vi "Read Measurement (FM Demodulation).vi"(0 "VISA resource name":refnum<visa-resource-name>, 11 "error in (no error)":errorcluster) -> (2 "Carrier Power (dBm)":dbl[](array[numeric]), 3 "Modulation Rate (Hz)":dbl[](array[numeric]), 4 "VISA resource name out":refnum<visa-resource-name>, 6 "Frequency Deviation (Hz)":dbl[](array[numeric]), 8 "SINAD (dB)":dbl[](array[numeric]), 10 "THD (dB)":dbl[](array[numeric]), 14 "Carrier Frequency Offset (Hz)":dbl[](array[numeric]), 15 "error out":errorcluster)   [LabVIEW 2022 SP3, in "Agilent N934X Series.lvlib"]
doc: "Reads the measurement result from the spectrum analyzer(FM Demodulation Measurement).\n\nNotes:\n\n(1) This VI is only applicable for N9321C, N9322C, N9323C, N9324C models.\n(2) User must use <B>Configure Measurement Type.vi</B> to change the mode to <B>Frequency Modulation</B> before using this VI."
uses:
  <instrlib>/Agilent N934X Series/Agilent N934X Series.lvlib
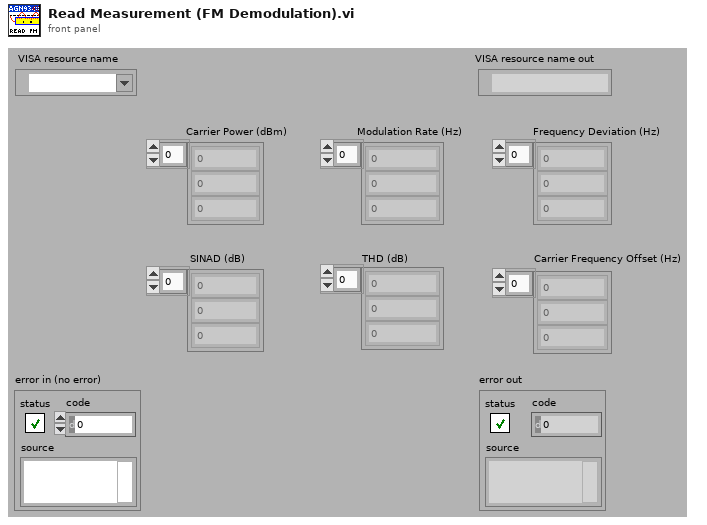
[diagram p1: front panel]
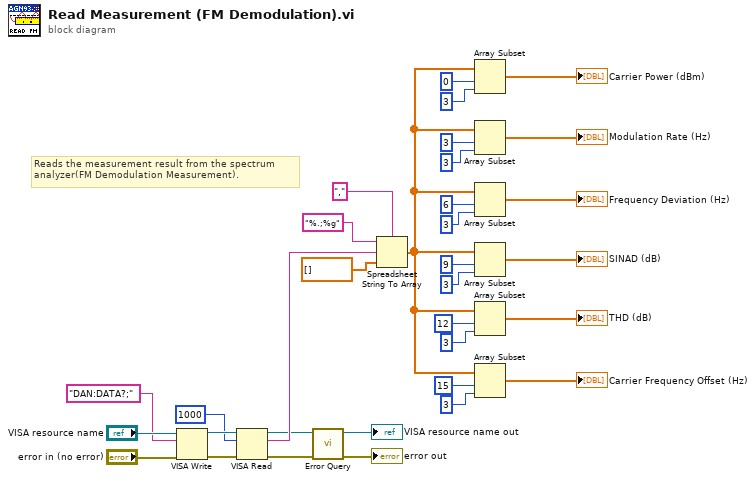
[diagram p0: block diagram]
diagram:
  # "Reads the measurement result from the spectrum \nanalyzer(FM Demodulation Measurement)."
  n1 = VISA Write(VISA resource name="VISA resource name", write buffer="DAN:DATA?;", error in (no error)="error in (no error)") -> (VISA resource name out=w32:refnum<visa-resource-name>, error out=w33:errorcluster)  [unwired: 1 out]
  n2 = VISA Read(VISA resource name=w32, byte count=u32 1000, error in (no error)=w33) -> (VISA resource name out=w6:refnum<visa-resource-name>, read buffer=w24:string, error out=w7:errorcluster)  [unwired: 1 out]
  n3 = call <instrlib>:"Error Query.vi"("error in (no error)"=w7, "VISA resource name"=w6) -> ("error out"=→"error out":errorcluster, "VISA resource name out"=→"VISA resource name out":refnum<visa-resource-name>)  [unwired: 6 in, 2 out]
  n4 = Spreadsheet String To Array(delimiter (Tab)=",", format string="%.;%g", spreadsheet string=w24, array type (2D Dbl)=dbl[] [] ("Measurement Data 2")) -> (array=w3:dbl[])
  n5 = Array Subset(array=w3, index=0, length=3) -> (→"Carrier Power (dBm)":dbl[])
  n6 = Array Subset(array=w3, index=3, length=3) -> (→"Modulation Rate (Hz)":dbl[])
  n7 = Array Subset(array=w3, index=6, length=3) -> (→"Frequency Deviation (Hz)":dbl[])
  n8 = Array Subset(array=w3, index=9, length=3) -> (→"SINAD (dB)":dbl[])
  n9 = Array Subset(array=w3, index=12, length=3) -> (→"THD (dB)":dbl[])
  n10 = Array Subset(array=w3, index=15, length=3) -> (→"Carrier Frequency Offset (Hz)":dbl[])
